vi "Get_Indicies_and_Number_of_Jumps-5_2.vi"(5 "[IN] Indicies for Jumps":i32[](array[numeric]), 8 "[IN] # of Track with\nFirst Problem Point":i32, 9 "[IN] Index of First Pro\nblem Point Inside Track":i32, 10 "[IN] Still connected\ntracks in group":T1) -> (3 "[OUT] Indexes for Jumps":i32[](array[numeric]))   [LabVIEW 2013]
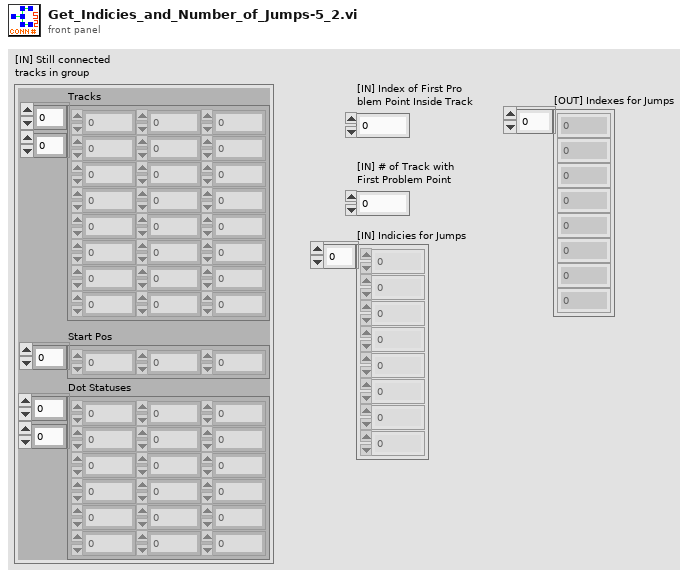
[diagram p1: front panel]
types:
  T1 = cluster{"Tracks":dbl[][], "Start Pos":i32[], "Dot Statuses":i16[][]}
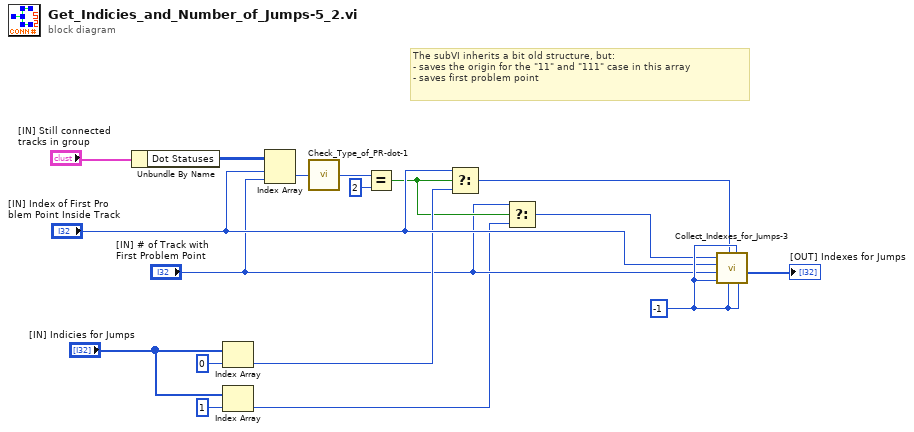
[diagram p0: block diagram]
diagram:
  w16 = -1 ("[IN] # Track with \nSecond Problem Point")
  # "The subVI inherits a bit old structure, but:  \n- saves the origin for the \"11\" and \"111\" case in this array\n- saves first problem point"
  n1 = Unbundle By Name("[IN] Still connected\ntracks in group") -> ("Dot Statuses"=w11:i16[][])
  n2 = Index Array(array="[IN] Indicies for Jumps", index=0) -> (element=w6:i32)
  n3 = Index Array(array="[IN] Indicies for Jumps", index=1) -> (element=w1:i32)
  n4 = Index Array(array=w11, index (row)="[IN] Index of First Pro\nblem Point Inside Track", index (col)="[IN] # of Track with\nFirst Problem Point") -> (element=w9:i16)
  n5 = call "Check_Type_of_PR-dot-1.vi"("[IN] dot status"=w9) -> ("[OUT] Type of\nproblem dot"=w8:i32)
  n6 = Equal?(x=w8, y=2) -> (x = y?=w5:bool)
  n7 = Select(t="[IN] Index of First Pro\nblem Point Inside Track", s=w5, f=w6) -> (s? t:f=w4:i32)
  n8 = Select(t="[IN] # of Track with\nFirst Problem Point", s=w5, f=w1) -> (s? t:f=w2:i32)
  n9 = call "Collect_Indexes_for_Jumps-3.vi"("[IN] # Track with \nThird Problem Point"=w16, "[IN] Index of Third\nProblem point"=w16, "[IN] # Track with \nSecond Problem Point"=w16, "[IN] Index of Point Be\nfore Problem (Origin)"=w4, "[IN] Index of Second\nProblem point"=w16, "[IN] # Track with First\nProblem Point"="[IN] # of Track with\nFirst Problem Point", "[IN] Index of First \nProblem Point"="[IN] Index of First Pro\nblem Point Inside Track", "[IN] # Track of Origin"=w2) -> ("[OUT] Indexes for Jumps"=→"[OUT] Indexes for Jumps":i32[])  [unwired: 3 in]
